vi "parse_itb.vi"(4 "error in":errorcluster, 7 "msg in":string="\u0000\u0000\u0000\u0000\u0000\u0000\u0000\u0000\u0000\u0000\u0000") -> (0 "error out":errorcluster, 2 "Navigator Inputs":T1, 3 "msg out":string)   [LabVIEW 2012]
doc: "Parses a message into ITB"
uses:
  std_msgs/subs/parse_bool_scalar.vi
  std_msgs/subs/parse_u8_scalar.vi
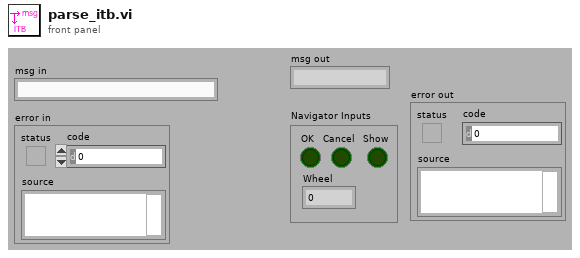
[diagram p1: front panel]
types:
  T1 = cluster{"OK":bool, "Cancel":bool, "Show":bool, "Wheel":u8}
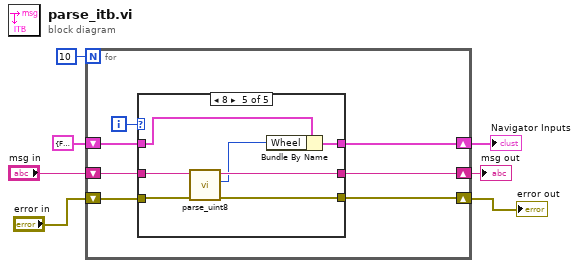
[diagram p0: block diagram]
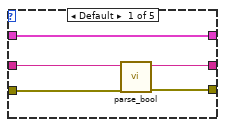
[diagram p2: hidden frame]
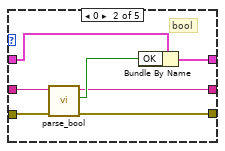
[diagram p3: hidden frame]
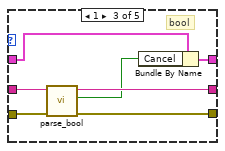
[diagram p4: hidden frame]
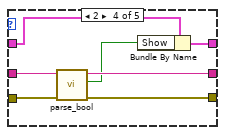
[diagram p5: hidden frame]
diagram:
  n1 = for {
    N: 10 -> [_]
    shift-right: [w12] -> w3
    shift-left: "msg in" -> [w13]
    shift-right: [w10] -> w6
    shift-left: T1 {"OK"=FALSE, "Cancel"=FALSE, "Show"=FALSE, "Wheel"=0} ("Navigator Inputs") -> [w11]
    shift-right: [w9] -> w1
    shift-left: "error in" -> [w8]
    i -> [w14]
    n2 = case shown="8" w14 {
      tunnel: [w17 w22 w30 w37 w44] -> w12
      tunnel: w13 -> [w18 w24 w31 w38 w45]
      tunnel: w11 -> [w19 w26 w33 w40 w47]
      tunnel: [w19 w25 w32 w39 w46] -> w10
      tunnel: [w16 w20 w28 w35 w42] -> w9
      tunnel: w8 -> [w15 w21 w27 w34 w41]
      frame Default {
        n3 = call-poly "parse_bool.vi"("error in"=w15, "msg in"=w18) -> ("error out"=w16:errorcluster, "msg out"=w17:string)  [unwired: 3 in, 1 out]
      }
      frame 0 {
        # "bool"
        n4 = call-poly "parse_bool.vi"("error in"=w21, "msg in"=w24) -> ("error out"=w20:errorcluster, "bool"=w23:bool, "msg out"=w22:string)  [unwired: 3 in]
        n5 = Bundle By Name(cluster=w26, "OK"=w23) -> (w25:T1)
      }
      frame 1 {
        # "bool"
        n6 = call-poly "parse_bool.vi"("error in"=w27, "msg in"=w31) -> ("error out"=w28:errorcluster, "bool"=w29:bool, "msg out"=w30:string)  [unwired: 3 in]
        n7 = Bundle By Name(cluster=w33, "Cancel"=w29) -> (w32:T1)
      }
      frame 2 {
        n8 = call-poly "parse_bool.vi"("error in"=w34, "msg in"=w38) -> ("error out"=w35:errorcluster, "bool"=w36:bool, "msg out"=w37:string)  [unwired: 3 in]
        n9 = Bundle By Name(cluster=w40, "Show"=w36) -> (w39:T1)
      }
      frame 8 {
        n10 = call-poly "parse_uint8.vi"("error in"=w41, "msg in"=w45) -> ("error out"=w42:errorcluster, "number"=w43:u8, "msg out"=w44:string)  [unwired: 3 in]
        n11 = Bundle By Name(cluster=w47, "Wheel"=w43) -> (w46:T1)
      }
    }
  }
  "Navigator Inputs" <- w6
  "msg out" <- w3
  "error out" <- w1
